vi "Run-plant.vi"(8 "error in (no error)":errorcluster, 11 "Plant VI path":path=path "../Plant1.vi") -> (0 "error out":errorcluster, 3 "reference out":refnum<vi>)   [LabVIEW 2016]
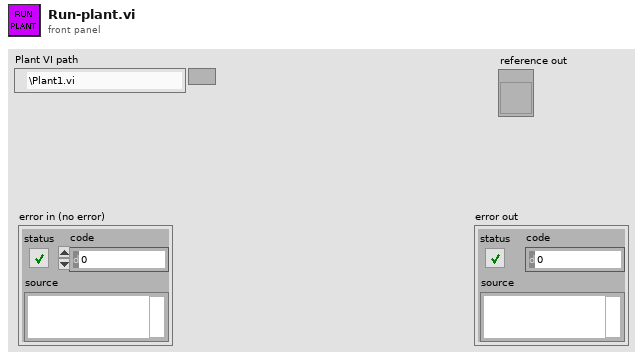
[diagram p1: front panel]
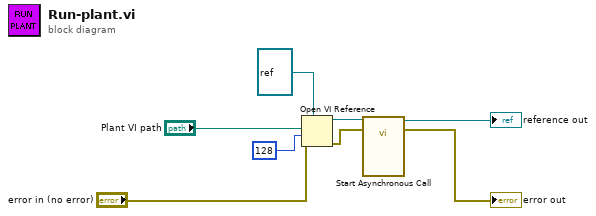
[diagram p0: block diagram]
diagram:
  n1 = Open VI Reference(type specifier VI Refnum (for type only)=refnum<vi> refnum, vi path="Plant VI path", options=128, error in (no error)="error in (no error)") -> (vi reference=w4:refnum<vi>, error out=w8:errorcluster)  [unwired: 2 in]
  n2 = call-by-ref "Start Asynchronous Call"(reference=w4, error in=w8) -> (reference out=→"reference out":refnum<vi>, error out=→"error out":errorcluster)  [unwired: 11 in, 1 out]
